vi "RWPrefCluster.vi"(7 "Task":enum16{"Read", "Write"}(ring), 8 "error in (no error)":errorcluster, 11 "Device In":T1={"Name"="", "BaseURL"="", "AppKey"="", "Headers"=["Content-Type:application/json"], "Timeout"=10000, "Identifier"="", "Password"="", "Comments"="", "Handle"=0, "# Handles"=0}) -> (0 "error out":errorcluster, 3 "Device Out":T1={"Name"="", "BaseURL"="", "AppKey"="", "Headers"=["Content-Type:application/json"], "Timeout"=10000, "Identifier"="", "Password"="", "Comments"="", "Handle"=0, "# Handles"=0})   [LabVIEW 2016]
uses:
  Device.ctl
panel:
  out "text":string
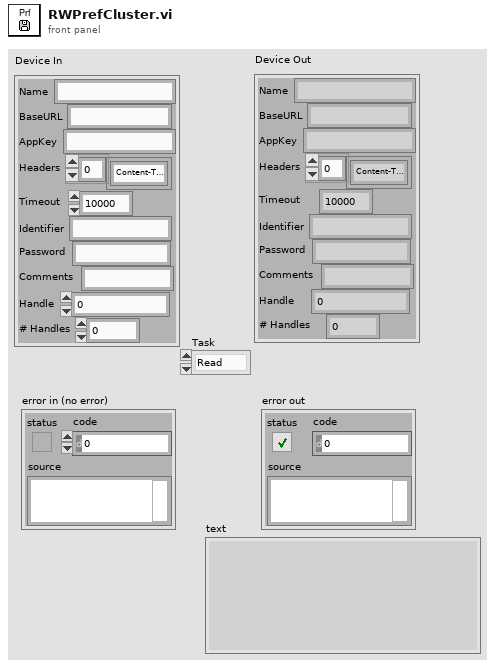
[diagram p1: front panel]
types:
  T1 = typedef "Device.ctl" = cluster{"Name":string, "BaseURL":string, "AppKey":string, "Headers":string[], "Timeout":i32, "Identifier":string, "Password":string, "Comments":string, "Handle":u32, "# Handles":i32}
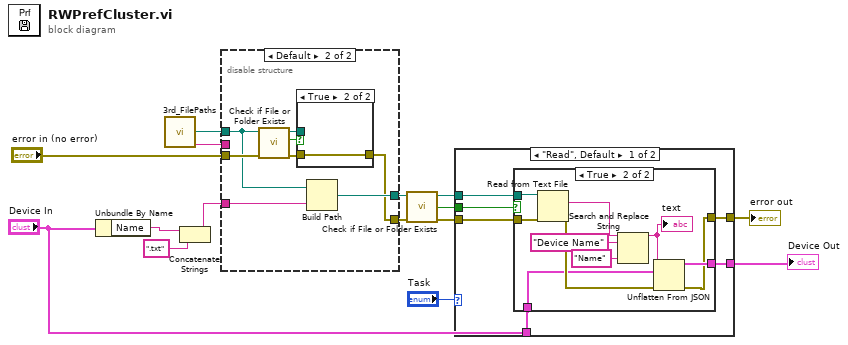
[diagram p0: block diagram]
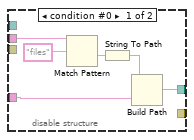
[diagram p2: hidden frame]
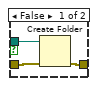
[diagram p3: hidden frame]
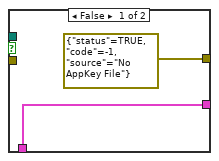
[diagram p4: hidden frame]
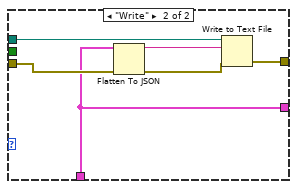
[diagram p5: hidden frame]
diagram:
  n1 = Unbundle By Name("Device In") -> ("Name"=w7:string)
  n2 = call "3rd_FilePaths.vi"() -> ("AppFiles on RIO"=w1:string, "AppKey Files"=w2:path)  [unwired: 9 in, 1 out]
  n3 = Concatenate Strings(w7, ".txt" ("string")) -> (w14:string)
  n4 = disable-structure shown="Default" {
    disable-tunnel: w14 -> [w17 w29]
    disable-tunnel: [w16 w28] -> w13
    disable-tunnel: "error in (no error)" -> [_ w25]
    disable-tunnel: [_ w23] -> w3
    disable-tunnel: w2 -> [_ w22]
    disable-tunnel: w1 -> [w21 _]
    frame condition #0 {
      n5 = Match Pattern(string=w21, regular expression="files" ("string")) -> (after substring=w19:string)  [unwired: 1 in, 3 out]
      n6 = String To Path(string=w19) -> (path=w18:path)
      n7 = Build Path(base path=w18, name or relative path=w17) -> (appended path=w16:path)
    }
    frame condition #1 (active) {
      n8 = call <vilib>:"Check if File or Folder Exists.vi"("error in (no error)"=w25, "path"=w22) -> ("error out"=w24:errorcluster, "file or folder exists?"=w27:bool, "dup path"=w26:path)  [unwired: 7 in]
      n9 = case shown="True" w27 {
        tunnel: w26 -> [w32 _]
        tunnel: w24 -> [w31 w33]
        tunnel: [w30 w33] -> w23
        frame False {
          n10 = Create Folder(path (use dialog)=w32, error in=w31) -> (error out=w30:errorcluster)  [unwired: 1 in, 2 out]
        }
        frame True {
        }
      }
      n11 = Build Path(base path=w22, name or relative path=w29) -> (appended path=w28:path)
    }
  }
  n12 = call <vilib>:"Check if File or Folder Exists.vi"("error in (no error)"=w3, "path"=w13) -> ("error out"=w11:errorcluster, "file or folder exists?"=w8:bool, "dup path"=w12:path)  [unwired: 7 in]
  n13 = case shown="\"Read\", Default" "Task" {
    tunnel: w12 -> [w38 w57]
    tunnel: w11 -> [w39 w55]
    tunnel: [w37 w53] -> w9
    tunnel: w8 -> [w36 _]
    tunnel: [w35 w52] -> w5
    tunnel: "Device In" -> [w34 w52]
    frame "Read", Default {
      n14 = case shown="True" w36 {
        tunnel: w39 -> [_ w51]
        tunnel: w38 -> [_ w50]
        tunnel: [errorcluster {"status"=TRUE, "code"=-1, "source"="No AppKey File"} ("error out") w46] -> w37
        tunnel: [w40 w47] -> w35
        tunnel: w34 -> [w40 w48]
        frame False {
        }
        frame True {
          n15 = Read from Text File(file (use dialog)=w50, error in=w51) -> (text=w45:string, error out=w49:errorcluster)  [unwired: 2 in, 2 out]
          n16 = Search and Replace String(input string=w45, search string="Device Name", replace string="Name" ("replace string (\"\")")) -> (result string=w42:string)  [unwired: 5 in, 3 out]
          "text" <- w42
          n17 = Unflatten From JSON(JSON string=w42, type and defaults=w48, error in (no error)=w49) -> (value=w47:T1, error out=w46:errorcluster)  [unwired: 4 in]
        }
      }
    }
    frame "Write" {
      n18 = Flatten To JSON(anything=w52, error in (no error)=w55) -> (JSON string=w56:string, 11:w54:errorcluster)  [unwired: 1 in]
      n19 = Write to Text File(file (use dialog)=w57, text=w56, error in=w54) -> (error out=w53:errorcluster)  [unwired: 1 in, 2 out]
    }
  }
  "error out" <- w9
  "Device Out" <- w5
